vi "Main_maszyna.vi"() -> ()   [LabVIEW 2013]
doc: "Use this template to build a standard state machine design pattern. Each state executes code and determines which state to transition to. Contrast this design pattern with the User Interface Event Handler pattern, in which code executes in response to user actions. Contrast this design pattern also with the Queued Message Handler pattern, in which each message handling code can queue zero or more new messages.\nNote: This template does not contain the most recent programming guidelines recommended by National Instruments. For a complete, project-based implementation of the Standard State Machine pattern, use the Create Project dialog box instead of this template."
uses:
  inne pliki/Stany.ctl
  inne pliki/Params.ctl
  inne pliki/Data.ctl
  inne pliki/Akcje czas FVG.ctl
  <vilib>/Utility/error.llb/DialogType.ctl
  <vilib>/Utility/file.llb/Write To Spreadsheet File (DBL).vi
panel:
  in  "path out 2":path
  out "path out":path
  in  "Generuj (F)":bool
  in  "Error?":bool
  out "Czas do końca pomiaru":dbl
  in  "bStopPomiar":bool
  out "Warning text":string
  out "Warning":bool
  in  "Temp limits":T1={"Max (25)"=22.0, "Min (0)"=0.0}
  out "Waveform Chart":cluster{"Temperatura":dbl, "Średnia":dbl}(graph)
  in  "Akcje":T2
  out "Stan aktualny":T3
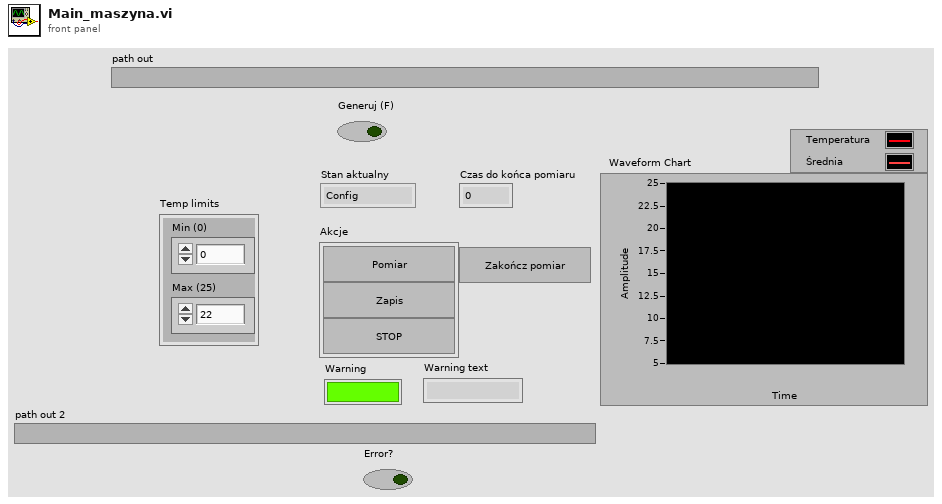
[diagram p1: front panel]
types:
  T1 = typedef "Params.ctl" = cluster{"Max (25)":dbl, "Min (0)":dbl}
  T2 = cluster{"bPomiar":bool, "bZapis":bool, "bSTOP":bool}
  T3 = typedef "Stany.ctl" = enum16{"Config", "IDLE", "Measure", "Analyze", "Display", "STOP", "Save", "Error", "Error end"}
  T4 = typedef "Data.ctl" = cluster{"Temperatura":dbl, "Średnia":dbl, "Warning":bool, "Warning text ":string, "Temp limits":T1, "Temp Array":dbl[], "Sternia Array":dbl[]}
  T5 = typedef "Akcje czas FVG.ctl" = enum16{"Reset", "Wait"}
  T6 = typedef "DialogType.ctl" = u16
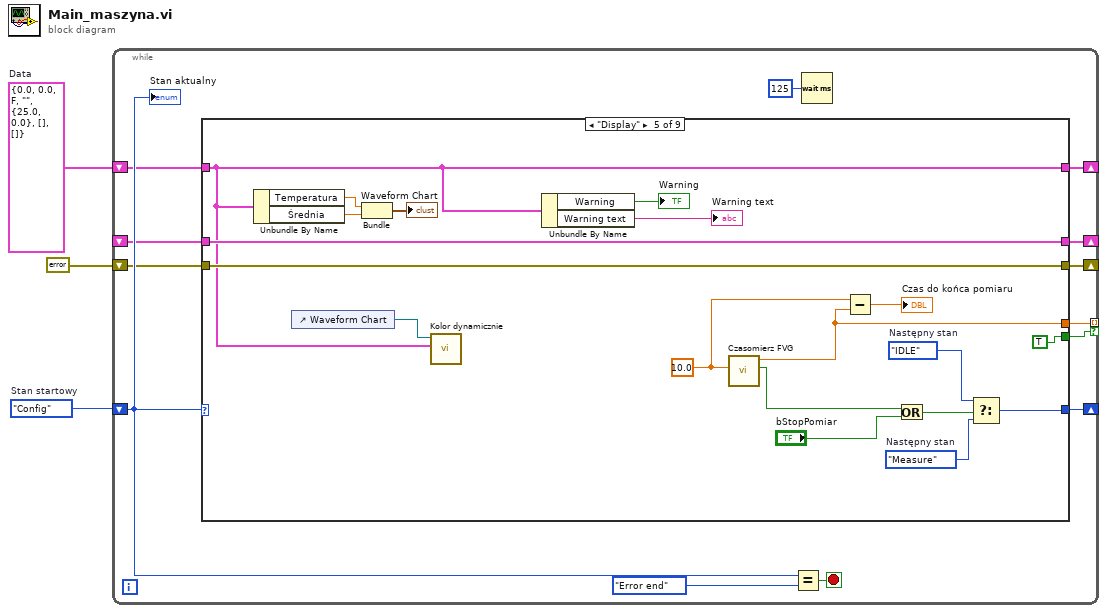
[diagram p0: block diagram]
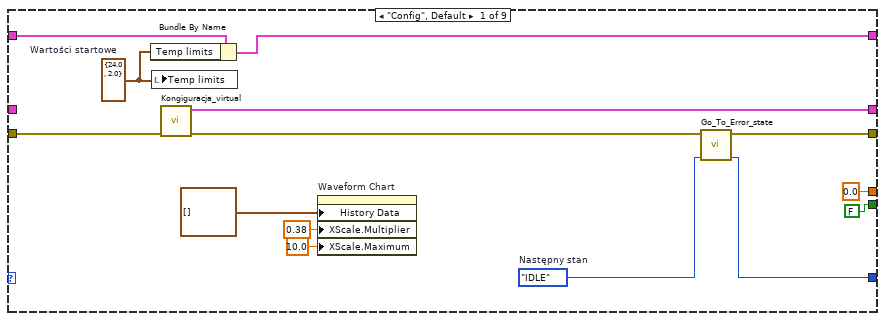
[diagram p2: hidden frame]
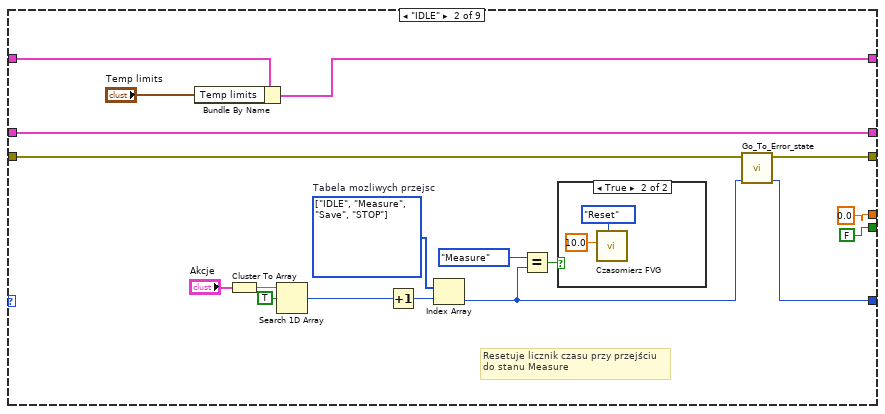
[diagram p3: hidden frame]
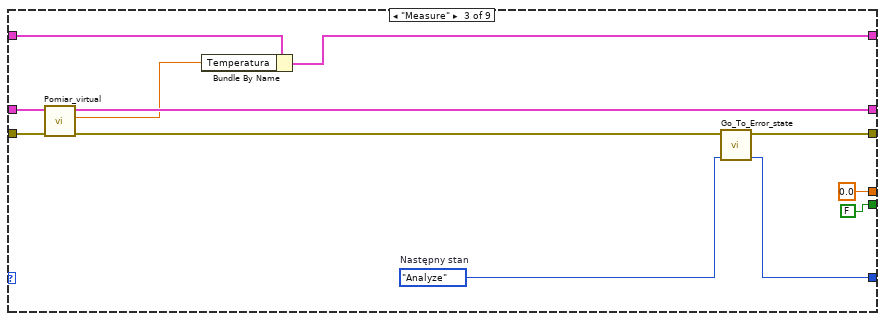
[diagram p5: hidden frame]
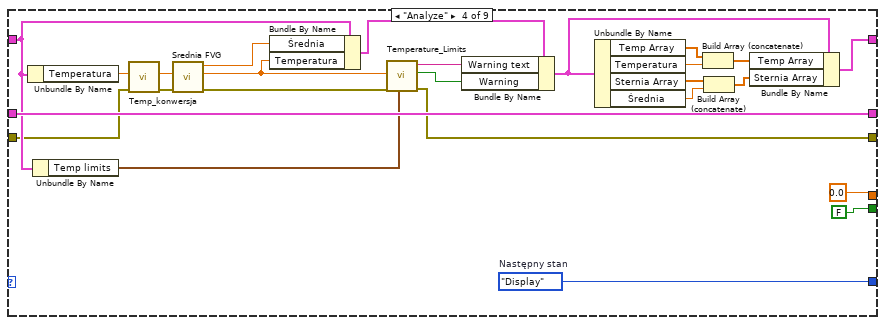
[diagram p6: hidden frame]
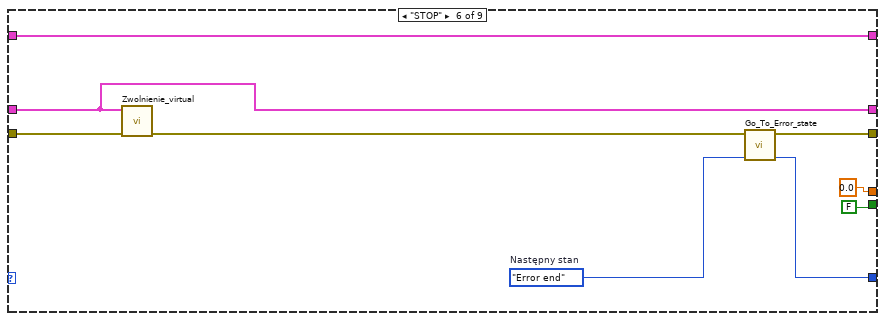
[diagram p7: hidden frame]
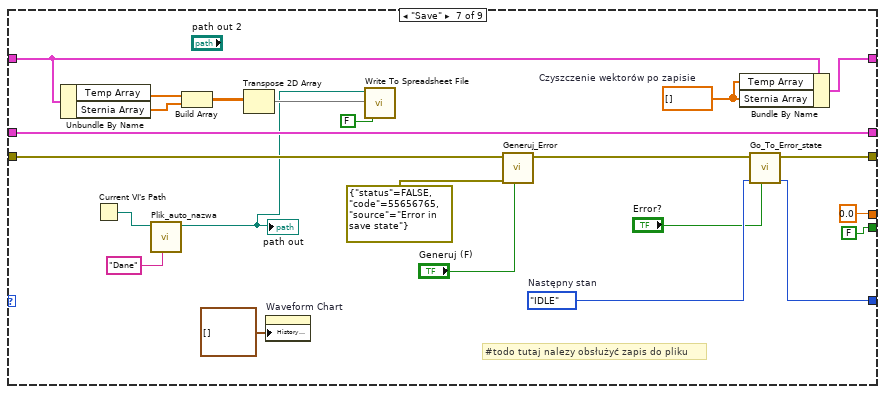
[diagram p8: hidden frame]
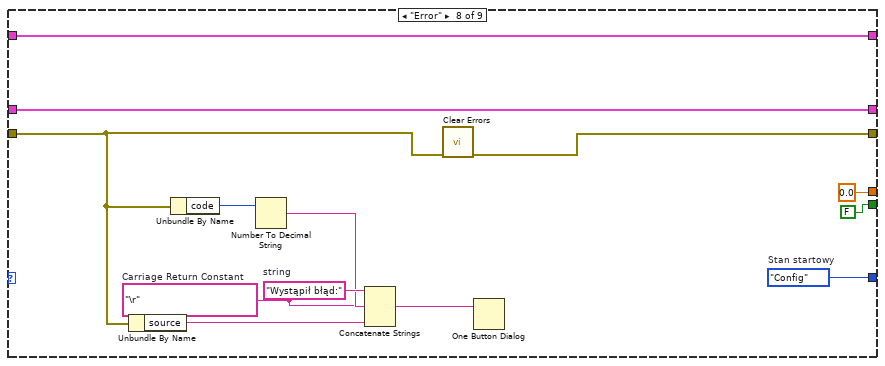
[diagram p9: hidden frame]
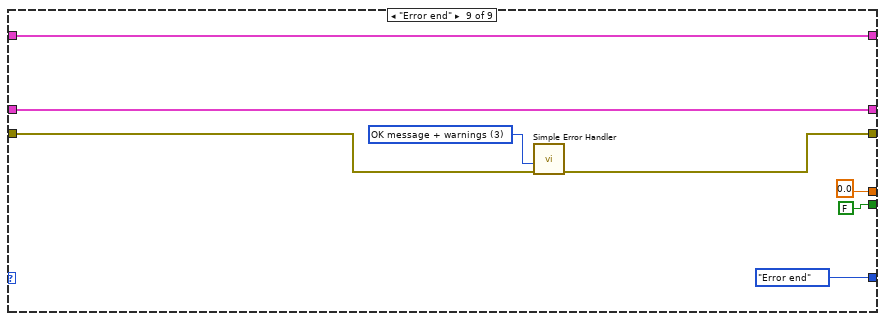
[diagram p10: hidden frame]
diagram:
  w2 = T4 {"Temperatura"=0.0, "Średnia"=0.0, "Warning"=FALSE, "Warning text "="", "Temp limits"={"Max (25)"=25.0, "Min (0)"=0.0}, "Temp Array"=[], "Sternia Array"=[]}  # Data
  w3 = Stany."Config"  # Stan startowy
  n1 = while {
    shift-right: [w14] -> _
    shift-left: w3 -> [w15]
    shift-right: [w10] -> _
    shift-left: w2 -> [w11]
    shift-right: [w9] -> _
    shift-left: _ -> [w8]
    shift-right: [w7] -> _
    shift-left: errorcluster {"status"=FALSE, "code"=0, "source"=""} ("error out") -> [w6]
    tunnel: [w5] -> _ mode=indexing if=w4
    stop <- w16 stop-if-true
    n2 = case shown="\"Display\"" w15 {
      tunnel: [w23 w33 w53 w87 w99 w109 w134 w148 Stany."Error end" ("Stan startowy")] -> w14
      tunnel: w11 -> [w28 w40 w58 w83 w92 w115 w128 w151 w159]
      tunnel: [w27 w39 w57 w65 w92 w115 w137 w151 w159] -> w10
      tunnel: [w30 w42 w61 w86 w106 w113 w138 w150 w158] -> w9
      tunnel: w8 -> [_ w42 w62 w86 w106 w113 w138 w150 w158]
      tunnel: [w24 w36 w56 w78 w105 w112 w135 w149 w155] -> w7
      tunnel: w6 -> [w29 w35 w60 w79 w105 w114 w123 w141 w156]
      tunnel: [0.0 ("Elapsed Time") 0.0 ("Elapsed Time") 0.0 ("Elapsed Time") 0.0 ("Elapsed Time") w90 0.0 ("Elapsed Time") 0.0 ("Elapsed Time") 0.0 ("Elapsed Time") 0.0 ("Elapsed Time")] -> w5
      tunnel: [FALSE FALSE FALSE FALSE TRUE FALSE FALSE FALSE FALSE] -> w4
      frame "Config", Default {
        w26 = T1 {"Max (25)"=24.0, "Min (0)"=2.0}  # Wartości startowe
        w22 = Stany."IDLE"  # Następny stan
        n3 = Bundle By Name(cluster=w28, "Temp limits"=w26) -> (w27:T4)
        n4 = local write "Temp limits"(w26) -> ()
        n5 = call "Kongiguracja_virtual.vi"("error in (no error)"=w29) -> ("error out"=w25:errorcluster, "Reference out"=w30:cluster{"Numeric":dbl, "Boolean":bool})  [unwired: 9 in]
        n6 = property on="Waveform Chart" class="WFChart (strict)"("History Data"=cluster{"Temperatura":dbl, "Średnia":dbl}[] [], "XScale.Multiplier"=0.38 ("X Scale.Offset and Multiplier:Multiplier"), "XScale.Maximum"=10.0 ("X Scale.Range:Maximum")) -> ()  [unwired: 2 in, 2 out]
        n7 = call "Go_To_Error_state.vi"("Następny stan in"=w22, "error in (no error)"=w25) -> ("Następny stan out"=w23:T3, "error out"=w24:errorcluster)  [unwired: 8 in]
      }
      frame "IDLE" {
        w43 = T3[] [enum."IDLE", enum."Measure", enum."Save", enum."STOP"] items=["Config", "IDLE", "Measure", "Analyze", "Display", "STOP", "Save", "Error", "Error end"]  # Tabela mozliwych przejsc
        # "Resetuje licznik czasu przy przejściu\ndo stanu Measure"
        n8 = Bundle By Name(cluster=w40, "Temp limits"="Temp limits") -> (w39:T4)
        n9 = Cluster To Array(cluster="Akcje") -> (array=w47:bool[])
        n10 = Search 1D Array(1D array=w47, element=TRUE) -> (index of element=w45:i32)  [unwired: 1 in]
        n11 = Increment(x=w45) -> (x+1=w44:i32)
        n12 = Index Array(array=w43, index=w44) -> (element=w34:T3)
        n13 = Equal?(x=Stany."Measure" ("Następny stan"), y=w34) -> (x = y?=w38:bool)
        n14 = case shown="True" w38 {
          frame False {
          }
          frame True {
            n15 = call "Czasomierz FVG.vi"("Akcja (Wait)"=Akcje_czas_FVG."Reset", "Czas (s)"=10.0) -> ()  [unwired: 7 in, 3 out]
          }
        }
        n16 = call "Go_To_Error_state.vi"("Następny stan in"=w34, "error in (no error)"=w35) -> ("Następny stan out"=w33:T3, "error out"=w36:errorcluster)  [unwired: 8 in]
      }
      frame "Measure" {
        w54 = Stany."Analyze"  # Następny stan
        n17 = call "Pomiar_virtual.vi"("error in (no error)"=w60, "Reference in"=w62) -> ("error out"=w55:errorcluster, "out"=w59:dbl, "Reference out"=w61:cluster{"Numeric":dbl, "Boolean":bool})  [unwired: 7 in]
        n18 = Bundle By Name(cluster=w58, "Temperatura"=w59) -> (w57:T4)
        n19 = call "Go_To_Error_state.vi"("Następny stan in"=w54, "error in (no error)"=w55) -> ("Następny stan out"=w53:T3, "error out"=w56:errorcluster)  [unwired: 8 in]
      }
      frame "Analyze" {
        w87 = Stany."Display"  # Następny stan
        n20 = Unbundle By Name(w83) -> ("Temperatura"=w85:dbl)
        n21 = Unbundle By Name(w83) -> ("Temp limits"=w84:T1)
        n22 = call "Temp_konwersja.vi"("error in (no error)"=w79, "Temp in"=w85) -> ("error out"=w77:errorcluster, "Temp out"=w76:dbl)  [unwired: 8 in]
        n23 = call "Srednia FVG.vi"("error in (no error)"=w77, "temperatura in"=w76) -> ("error out"=w75:errorcluster, "temperatura out"=w74:dbl, "średnia out"=w73:dbl)  [unwired: 7 in]
        n24 = Bundle By Name(cluster=w83, "Średnia"=w73, "Temperatura"=w74) -> (w80:T4)
        n25 = call "Temperature_Limits.vi"("Temp limits"=w84, "error in (no error)"=w75, "TEMP"=w74) -> ("error out"=w78:errorcluster, "Warning"=w81:bool, "Warning Text"=w82:string)  [unwired: 6 in]
        n26 = Bundle By Name(cluster=w80, "Warning text"=w82, "Warning"=w81) -> (w66:T4)
        n27 = Unbundle By Name(w66) -> ("Temp Array"=w72:dbl[], "Temperatura"=w71:dbl, "Sternia Array"=w70:dbl[], "Średnia"=w69:dbl)
        n28 = Build Array (concatenate)(w72, w71) -> (w68:dbl[])
        n29 = Build Array (concatenate)(w70, w69) -> (w67:dbl[])
        n30 = Bundle By Name(cluster=w66, "Temp Array"=w68, "Sternia Array"=w67) -> (w65:T4)
      }
      frame "Display" {
        w94 = 10.0 ("Czas (s)")
        w98 = Stany."Measure"  # Następny stan
        w100 = Stany."IDLE"  # Następny stan
        n31 = Unbundle By Name(w92) -> ("Temperatura"=w91:dbl, "Średnia"=w104:dbl)
        n32 = control-ref of="Waveform Chart"() -> (w88:refnum<vi>)
        n33 = Bundle("Temperatura"=w91, "Średnia"=w104) -> (→"Waveform Chart":cluster{"Temperatura":dbl, "Średnia":dbl})  [unwired: 1 in]
        n34 = call "Kolor dynamicznie.vi"("Data"=w92, "WaveformChart in"=w88) -> ()  [unwired: 9 in, 1 out]
        n35 = Unbundle By Name(w92) -> ("Warning"=→"Warning":bool, "Warning text"=→"Warning text":string)
        n36 = call "Czasomierz FVG.vi"("Czas (s)"=w94) -> ("Elapsed?"=w95:bool, "Elapsed Time"=w90:dbl)  [unwired: 8 in, 1 out]
        n37 = Subtract(x=w94, y=w90) -> (x-y=→"Czas do końca pomiaru":dbl)
        n38 = Or(x=w95, y="bStopPomiar") -> (x .or. y?=w97:bool)
        n39 = Select(t=w100, s=w97, f=w98) -> (s? t:f=w99:T3)
      }
      frame "STOP" {
        w110 = Stany."Error end"  # Następny stan
        n40 = call "Zwolnienie_virtual.vi"("error in (no error)"=w114, "Reference in"=w113) -> ("error out"=w111:errorcluster)  [unwired: 9 in]
        n41 = call "Go_To_Error_state.vi"("Następny stan in"=w110, "error in (no error)"=w111) -> ("Następny stan out"=w109:T3, "error out"=w112:errorcluster)  [unwired: 8 in]
      }
      frame "Save" {
        w136 = dbl[] []  # Czyszczenie wektorów po zapisie
        w133 = Stany."IDLE"  # Następny stan
        # "#todo tutaj nalezy obsłużyć zapis do pliku"
        n42 = Unbundle By Name "Unbundle By Name"(w128) -> ("Temp Array"=w127:dbl[], "Sternia Array"=w126:dbl[])
        n43 = Current VI's Path() -> (path=w121:path)
        n44 = call "Plik_auto_nazwa.vi"("Nazwa in"="Dane", "path in"=w121) -> ("path out"=w119:path)  [unwired: 8 in, 1 out]
        "path out" <- w119
        n45 = Build Array "Build Array"(w127, w126) -> (w125:dbl[][])
        n46 = Transpose 2D Array(2D array=w125) -> (transposed array=w124:dbl[][])
        n47 = property on="Waveform Chart" class="WFChart (strict)"("History Data"=cluster{"Temperatura":dbl, "Średnia":dbl}[] []) -> ()  [unwired: 2 in, 2 out]
        n48 = call-poly <vilib>:"Write To Spreadsheet File.vi"("append to file? (new file:F)"=FALSE, "2D data"=w124, "file path (dialog if empty)"=w119) -> ()  [unwired: 5 in, 1 out]
        n49 = call "Generuj_Error.vi"("Generuj (F)"="Generuj (F)", "Generator"=errorcluster {"status"=FALSE, "code"=55656765, "source"="Error in save state"}, "error in (no error)"=w123) -> ("error out"=w131:errorcluster)  [unwired: 8 in]
        n50 = Bundle By Name(cluster=w128, "Temp Array"=w136, "Sternia Array"=w136) -> (w137:T4)
        n51 = call "Go_To_Error_state.vi"("GoTo Error (F)"="Error?", "Następny stan in"=w133, "error in (no error)"=w131) -> ("Następny stan out"=w134:T3, "error out"=w135:errorcluster)  [unwired: 7 in]
      }
      frame "Error" {
        w144 = "\r"  # Carriage Return Constant
        w146 = "Wystąpił błąd:"  # string
        w148 = Stany."Config"  # Stan startowy
        n52 = Unbundle By Name(w141) -> ("source"=w142:string)
        n53 = Unbundle By Name(w141) -> ("code"=w147:i32)
        n54 = Number To Decimal String(number=w147) -> (decimal integer string=w145:string)  [unwired: 1 in]
        n55 = Concatenate Strings "Concatenate Strings"(w146, w144, w145, w144, w142) -> (w143:string)
        n56 = call <vilib>:"Clear Errors.vi"("error in (no error)"=w141) -> ("error out"=w149:errorcluster)  [unwired: 6 in]
        n57 = One Button Dialog(message=w143) -> ()  [unwired: 1 in, 1 out]
      }
      frame "Error end" {
        w154 = T6 3 items=["no dialog", "OK message", "continue or stop message", "OK message + warnings", "continue/stop + warnings"] ("type of dialog (OK msg:1)")
        n58 = call <vilib>:"Simple Error Handler.vi"("type of dialog (OK msg:1)"=w154, "error in (no error)"=w156) -> ("error out"=w155:errorcluster)  [unwired: 3 in, 4 out]
      }
    }
    n59 = Equal?(x=w15, y=Stany."Error end" ("Stan startowy")) -> (x = y?=w16:bool)
    n60 = Wait (ms)(milliseconds to wait=u32 125) -> ()  [unwired: 1 out]
    "Stan aktualny" <- w15
  }
